vi "Create_Default_Destinations.vi"(8 "error in (no error)":errorcluster, 9 "Destination Name":string, 10 "Destination Path":path, 11 "AB_SourceDistribution in":refnum<class "AB_SourceDistribution.lvclass">) -> (0 "error out":errorcluster, 2 "default dests":refnum<class "AB_Destination.lvclass">[](array[class]), 3 "AB_SourceDistribution out":refnum<class "AB_SourceDistribution.lvclass">)   [LabVIEW 2020, in "AB_SourceDistribution.lvclass"]
uses:
  <vilib>/AppBuilder/AB_Classes/SourceDistribution/AB_SourceDistribution.lvclass
  <vilib>/AppBuilder/AB_Classes/Destination/AB_Destination.lvclass
  <vilib>/AppBuilder/AB_Classes/Destination/AB_Destination.ctl
  <resource>/Framework/Providers/Common/provcom_StringGlobals.vi
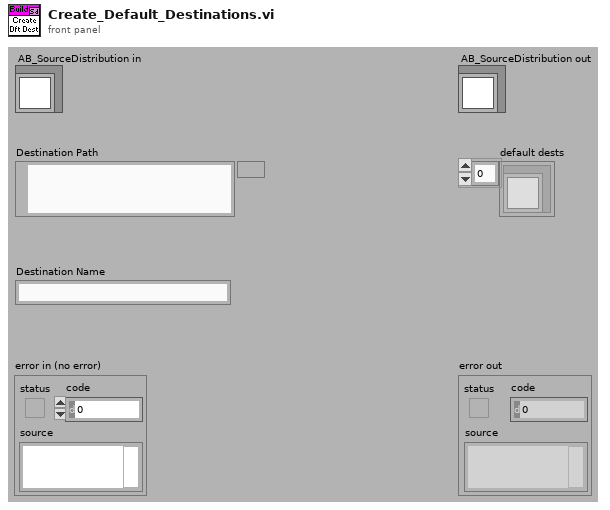
[diagram p1: front panel]
types:
  T1 = typedef "AB_Destination.ctl" = cluster{"destName":string, "path":path, "libraryName":string, "preserveHierarchy":bool, "eng_inBuild":bool, "eng_libraryReference":refnum<vi>, "eng_restictAddToNewLibrary":bool}
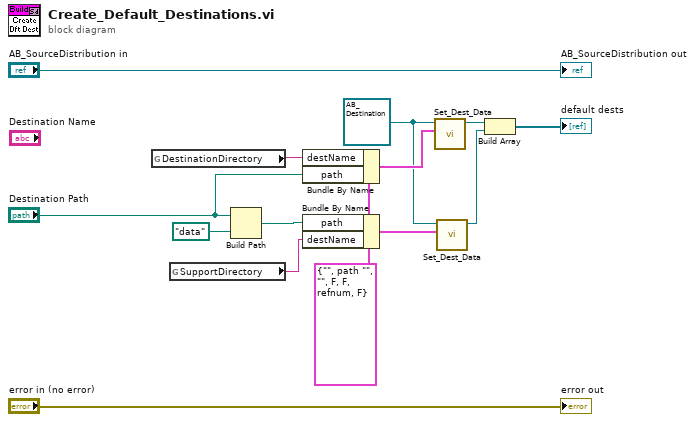
[diagram p0: block diagram]
diagram:
  w5 = T1 {"destName"="", "path"=path "", "libraryName"="", "preserveHierarchy"=FALSE, "eng_inBuild"=FALSE, "eng_libraryReference"=refnum, "eng_restictAddToNewLibrary"=FALSE} ("destName")
  w7 = refnum<class "AB_Destination.lvclass"> refnum ("AB_Destination.lvclass")
  n1 = global read "provcom_StringGlobals.vi" "DestinationDirectory"() -> (w6:string)
  n2 = global read "provcom_StringGlobals.vi" "SupportDirectory"() -> (w8:string)
  n3 = Build Path(base path="Destination Path", name or relative path=path "data") -> (appended path=w10:path)
  n4 = Bundle By Name(cluster=w5, "destName"=w6, "path"="Destination Path") -> (w12:T1)
  n5 = Bundle By Name(cluster=w5, "path"=w10, "destName"=w8) -> (w9:T1)
  n6 = call <vilib>:"Set_Dest_Data.vi"("destName"=w12, "Class in"=w7) -> ("Class out"=w13:refnum<class "AB_Destination.lvclass">)  [unwired: 1 in, 8 out]
  n7 = call <vilib>:"Set_Dest_Data.vi"("destName"=w9, "Class in"=w7) -> ("Class out"=w11:refnum<class "AB_Destination.lvclass">)  [unwired: 1 in, 8 out]
  n8 = Build Array(w13, w11) -> (→"default dests":refnum<class "AB_Destination.lvclass">[])
  "error out" <- "error in (no error)"
  "AB_SourceDistribution out" <- "AB_SourceDistribution in"
